vi "Measure vs B2Dv11.vi"() -> ()   [LabVIEW 2009]
doc: "This VI is an example operator panel.\n\nThe VI contains a table for the field values that may be configured manually, or loaded by checking the \"Prompt for File\" box. The data file should contain 3 columns of data, with each column delimited by a tab character.\n\nBefore the VI is executed, set the desired field units and coordinate system. Once the VI is started, follow the directions in the STATUS indicator to operate. Once a field value is achieved, it will be held indefinitely with no user intervention.\n\nThe present field is displayed in the selected units and coordinate system. The present field is queried once per second.\n\nIf a field point is specified that is outside the limits for the magnet, the VI will abort execution."
uses:
  <vilib>/Utility/file.llb/Read From Spreadsheet File (DBL).vi
panel:
  in  "Port Num- TRBridge":string="7"
  in  "GPIB SIM900":string="2"
  in  "TempSensor":bool=TRUE
  in  "AH":bool=TRUE
  in  "GPIB HP 2":string="13"
  in  "Wait between \nVectors":bool
  in  "Change\nPID\n(DetermineSIMPID.vi)":bool
  in  "Wait between \nVectors (ms)":u32=3000
  in  "X Axis":enum16{"B", "phi"}(ring)
  in  "Y Axis":T1(ring)=enum."HP (V)2"
  out "measured data":dbl[][](array[numeric])
  out "XY Graph":T2(graph)
  in  "Notes:":string="Datum: 16.01.12, Uhrzeit: 14:00, Sweep 0.15T/min,(measurevsB2Dv10.vi)), kapazitive Messung, leerer Sensor #1649_1, Referenzmessung, T=0.3K, Winkel 15° , optischer Probenstab, Gestell entfernt" caption="Notizen:"
  out "Messfile Refnum":refnum<file>
  in  "Measurement File":path=path "D:/UserData/Matthias/Messungen/#1649_leer/120116/120116_#1649_135deg_M1.txt"
  in  "Sample name:":string="#1649_1, leer"
  in  "HP 1":bool
  in  "GPIB HP":string="14"
  in  "HP 2":bool
  in  "LI 3":bool
  in  "GPIB L 3":string="8"
  in  "LI 2":bool
  in  "GPIB L 2":string="8"
  in  "LI 1":bool
  in  "GPIB L 1":string="8"
  out "Number of lines":i32=3
  in  "Operation":u16(ring)=1 items=["Stepwise", "Continous"]
  out "Ramp Rate along Vector (T/min)":dbl=0.2123426648592312 format="%.3f"
  out "Current Ramp Rate Z (T/min)":dbl=0.15014787650686168 format="%.3f"
  out "Current Ramp Rate Y (T/min)":dbl=0.15015 format="%.3f"
  in  "User defined Ramp Rate (T/min)":bool=TRUE
  in  "User defined Ramp Rate (T/min)":dbl=0.22 format="%.3f"
  in  "Z-Axis Communications Config":T3={"GPIB address"=22, "GPIB bus"=1, "connection ID"=refnum, "IP"="111.111.111.1", "Active Comm Interface"=0, "Serial Port"="", "Programmer Type"=0} {"Programmer Type" items=["Model 430", "Model 420"]; "Active Comm Interface" items=["TCP/IP (Model 430 Only)", "RS232", "IEEE488"]}
  in  "Max Ramp Rate - Y Axis (A/s)":dbl=0.055 format="%.3f"
  in  "Max Ramp Rate - Z Axis (A/s)":dbl=0.19 format="%.3f"
  in  "Magnitude Limit (kG)":dbl=45.1 format="%.3f"
  in  "Y-Axis Communications Config":T3={"GPIB address"=22, "GPIB bus"=1, "connection ID"=refnum, "IP"="111.111.111.2", "Active Comm Interface"=0, "Serial Port"="", "Programmer Type"=0} {"Programmer Type" items=["Model 430", "Model 420"]; "Active Comm Interface" items=["TCP/IP (Model 430 Only)", "RS232", "IEEE488"]}
  out "Cartesian Display (T)":T4={"Y-Axis Field (T)"=-1e-05, "Z-Axis Field (T)"=2.9999999999999997e-05} {"Z-Axis Field (T)" format="%.3f"; "Y-Axis Field (T)" format="%.3f"}
  in  "Starting index":i32=2
  in  "Normal color":u32(colorbox)=11711154
  in  "Highlight color":u32(colorbox)=16711680
  in  "Prompt for File?":bool
  out "Continue Execution?":bool=TRUE
  out "error out":T5
  in  "error in":T5
  out "STATUS":string="Zeroing vector."
  in  "Ramping Control":u16(ring)=4 items=["NEXT VECTOR", "RAMPING", "HOLDING", "PAUSE", "ZERO"]
  out "Cartesian Display (kG)":T6 {"Z-Axis Field (kG)" format="%.3f"; "Y-Axis Field (kG)" format="%.3f"}
  in  "Field Values":string[][](table)=[["4", "135"], ["-4", "135"], ["0", "0"]]
  out "Switch Heaters":bool=TRUE
  out "Polar Display (T)":T7={"q (degrees)"=315.0, "Field Magnitude (T)"=1.4142135623730951e-05} {"Field Magnitude (T)" format="%.3f"; "q (degrees)" format="%.3f"}
  out "Polar Display (kG)":T8 {"Field Magnitude (kG)" format="%.3f"; "q (degrees)" format="%.3f"}
  in  "Coordinate System":u16(ring)=1 items=["Cartesian", "Polar"]
  in  "Magnetic Field Units":u16(ring)=1 items=["kG", "Tesla"]
  # "kontinuirliche Messung mit PID off bei 0, geht nur im Cartesian mode!"
  # "Measurement Display"
  # "Measurement Settings"
  # "Magnet Settings"
  # "Max Ramp Rate z: 1.27 T/min\nMax Ramp Rate y: 0.17 T/min"
  # "Devices"
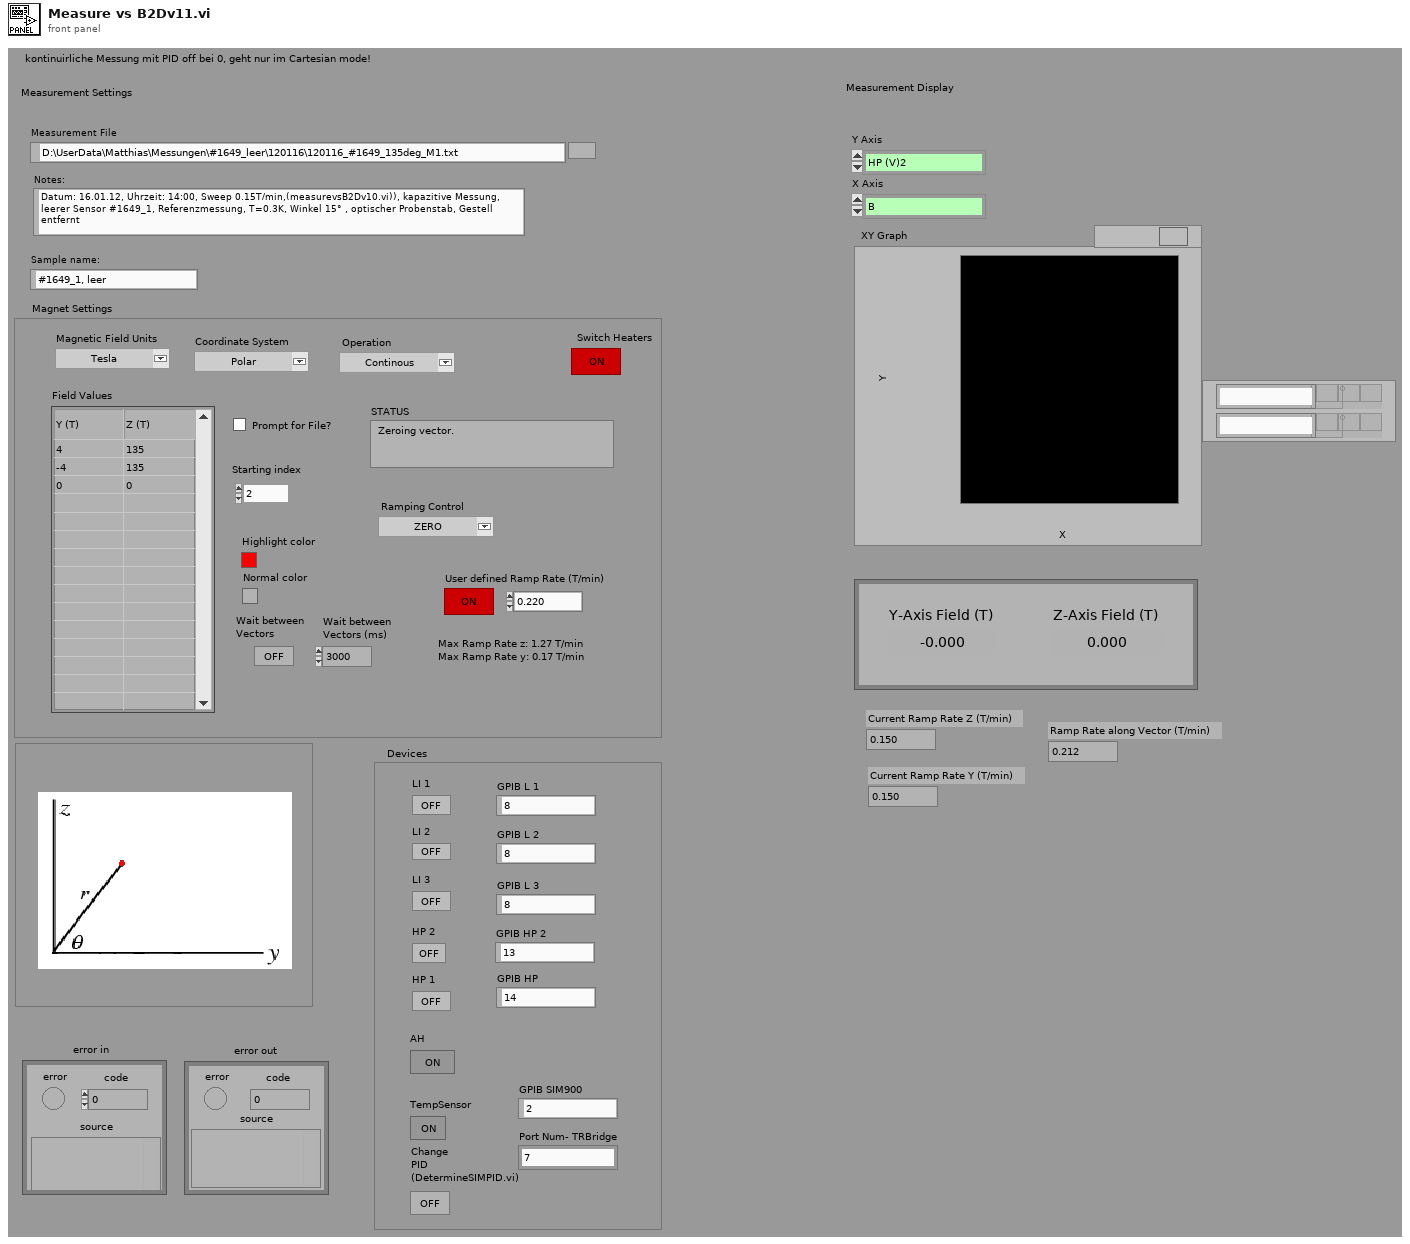
[diagram p1: front panel]
types:
  T1 = enum16{"B", "phi", "LI 1 Vx", "LI 1 Vy", "LI 2 Vx", "LI 2 Vy", "LI 3 Vx", "LI 3 Vy", "LI 4 Vx", "LI 4 Vy", "HP (V)", "HP (V)2", "AH C (pF)", "AH loss"}
  T2 = cluster{"measured data":dbl[], "measured data":dbl[]}
  T3 = cluster{"GPIB address":i16, "GPIB bus":i16, "connection ID":refnum<k5>, "IP":string, "Active Comm Interface":u16, "Serial Port":refnum<visa-resource-name>, "Programmer Type":u16}
  T4 = cluster{"Y-Axis Field (T)":dbl, "Z-Axis Field (T)":dbl}
  T5 = cluster{"error":bool, "code":i32, "source":string}
  T6 = cluster{"Y-Axis Field (kG)":dbl, "Z-Axis Field (kG)":dbl}
  T7 = cluster{"q (degrees)":dbl, "Field Magnitude (T)":dbl}
  T8 = cluster{"q (degrees)":dbl, "Field Magnitude (kG)":dbl}
  T9 = enum16{"", "RAMPING", "HOLDING", "PAUSED", "MANUAL UP", "MANUAL DOWN", "ZEROING CURRENT", "QUENCH DETECTED", "HEATING SWITCH"}
  T10 = enum16{"", "RAMPING", "HOLDING", "PAUSED", "MANUAL UP", "MANUAL DOWN", "ZEROING CURRENT", "QUENCH DETECTED", "HEATING SWITCH", "AT ZER0", "COOLING SWITCH"}
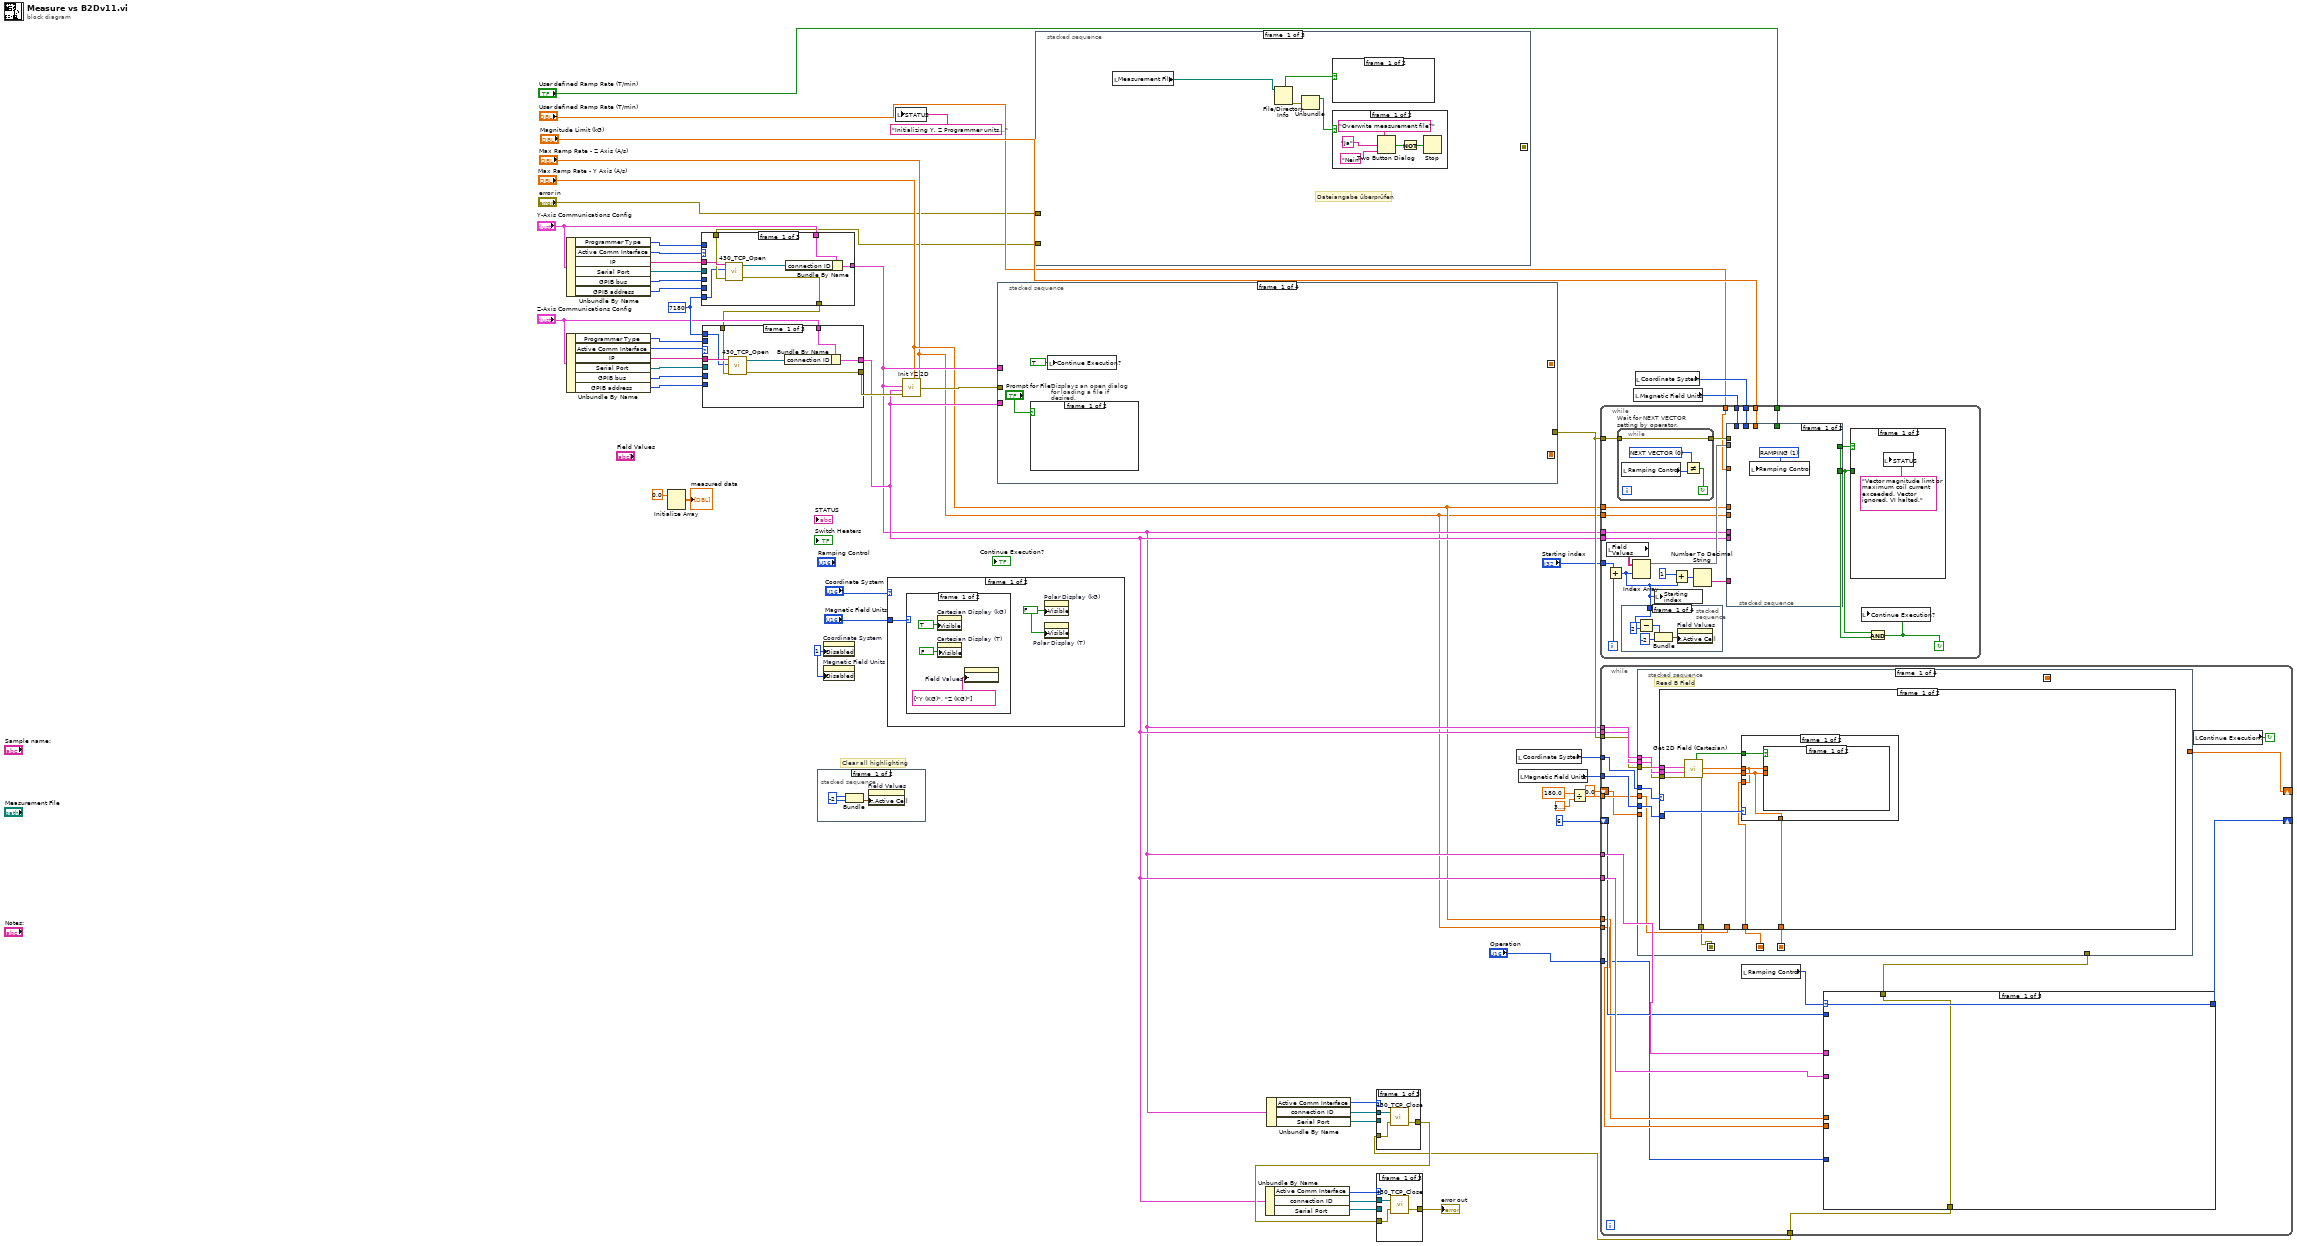
[diagram p0: block diagram]
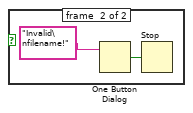
[diagram p3: hidden frame]
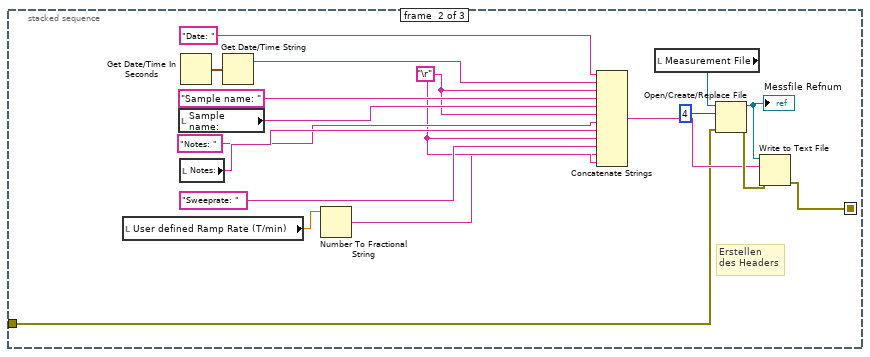
[diagram p4: hidden frame]
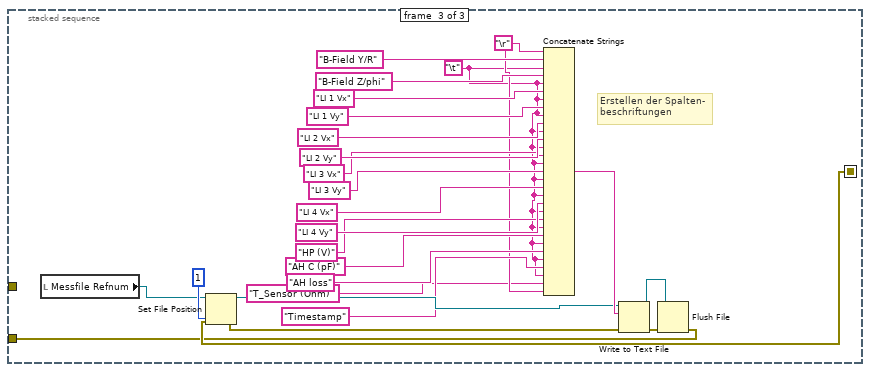
[diagram p5: hidden frame]
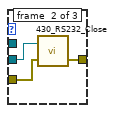
[diagram p6: hidden frame]
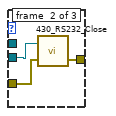
[diagram p8: hidden frame]
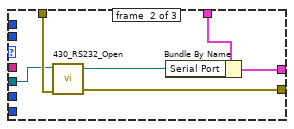
[diagram p10: hidden frame]
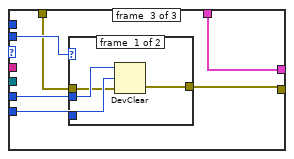
[diagram p11: hidden frame]
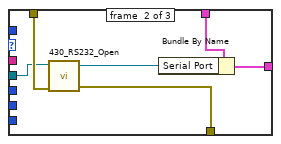
[diagram p13: hidden frame]
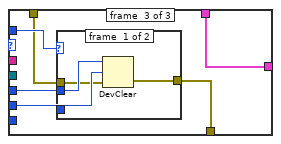
[diagram p14: hidden frame]
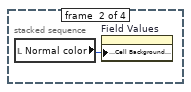
[diagram p16: hidden frame]
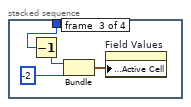
[diagram p17: hidden frame]
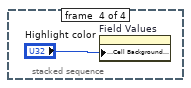
[diagram p18: hidden frame]
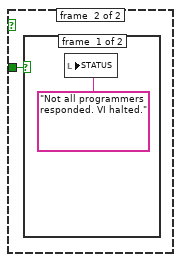
[diagram p19: hidden frame]
diagram:
  w39 = 7180 ("TCP Port")
  w52 = u8 1 ("Write Attribute")
  # "Clear all highlighting"
  n1 = Unbundle By Name("Z-Axis Communications Config") -> ("Programmer Type"=w15:u16, "Active Comm Interface"=w38:u16, "IP"=w35:string, "Serial Port"=w34:refnum<visa-resource-name>, "GPIB bus"=w14:i16, "GPIB address"=w13:i16)
  n2 = Unbundle By Name("Y-Axis Communications Config") -> ("Programmer Type"=w9:u16, "Active Comm Interface"=w37:u16, "IP"=w36:string, "Serial Port"=w33:refnum<visa-resource-name>, "GPIB bus"=w10:i16, "GPIB address"=w11:i16)
  n3 = Initialize Array(0.0 ("element")) -> (→"measured data":dbl[][])  [unwired: 2 in]
  n4 = stacked-sequence {
    frame #0 {
      w55 = -2
      n5 = Bundle(w55, w55) -> (w56:cluster{i32, i32})  [unwired: 1 in]
      n6 = property on="Field Values" class="Tbl (strict)"("Active Cell:Active Cell"=w56) -> ()  [unwired: 2 in, 2 out]
    }
    frame #1 {
      n7 = property on="Field Values" class="Tbl (strict)"("Active Cell:Cell Background Color"="Normal color") -> ()  [unwired: 2 in, 2 out]
    }
  }
  n8 = property on="Coordinate System" class="Ring (strict)"("Disabled"=w52) -> ()  [unwired: 2 in, 2 out]
  n9 = property on="Magnetic Field Units" class="Ring (strict)"("Disabled"=w52) -> ()  [unwired: 2 in, 2 out]
  n10 = case shown="0, Default" "Coordinate System" {
    tunnel: "Magnetic Field Units" -> [w59 w67]
    frame #0 {
      w58 = FALSE ("Write Attribute")
      (unwired) FALSE ("Write Attribute")
      (unwired) TRUE ("Write Attribute")
      n11 = case shown="1" w59 {
        frame #0 {
          n12 = property on="Cartesian Display (kG)" class="Cluster (strict)"("Visible"=TRUE ("Write Attribute")) -> ()  [unwired: 2 in, 2 out]
          n13 = property on="Cartesian Display (T)" class="Cluster (strict)"("Visible"=FALSE ("Write Attribute")) -> ()  [unwired: 2 in, 2 out]
          n14 = property on="Field Values" class="Tbl (strict)"("Column Header Strings[]"=string[] ["Y (KG)", "Z (KG)"] ("Write Attribute")) -> ()  [unwired: 2 in, 2 out]
        }
        frame #1 {
          n15 = property on="Cartesian Display (kG)" class="Cluster (strict)"("Visible"=FALSE ("Write Attribute")) -> ()  [unwired: 2 in, 2 out]
          n16 = property on="Cartesian Display (T)" class="Cluster (strict)"("Visible"=TRUE ("Write Attribute")) -> ()  [unwired: 2 in, 2 out]
          n17 = property on="Field Values" class="Tbl (strict)"("Column Header Strings[]"=string[] ["Y (T)", "Z (T)"] ("Write Attribute")) -> ()  [unwired: 2 in, 2 out]
        }
      }
      n18 = property on="Polar Display (kG)" class="Clust (strict)"("Visible"=w58) -> ()  [unwired: 2 in, 2 out]
      n19 = property on="Polar Display (T)" class="Clust (strict)"("Visible"=w58) -> ()  [unwired: 2 in, 2 out]
    }
    frame #1 {
      (unwired) FALSE ("Write Attribute")
      (unwired) TRUE ("Write Attribute")
      w66 = FALSE ("Write Attribute")
      n20 = case shown="1" w67 {
        frame #0 {
          n21 = property on="Polar Display (kG)" class="Clust (strict)"("Visible"=TRUE ("Write Attribute")) -> ()  [unwired: 2 in, 2 out]
          n22 = property on="Polar Display (T)" class="Clust (strict)"("Visible"=FALSE ("Write Attribute")) -> ()  [unwired: 2 in, 2 out]
          n23 = property on="Field Values" class="Tbl (strict)"("Column Header Strings[]"=string[] ["Mag. r (KG)", "Theta (deg)"] ("Write Attribute")) -> ()  [unwired: 2 in, 2 out]
        }
        frame #1 {
          n24 = property on="Polar Display (kG)" class="Clust (strict)"("Visible"=FALSE ("Write Attribute")) -> ()  [unwired: 2 in, 2 out]
          n25 = property on="Polar Display (T)" class="Clust (strict)"("Visible"=TRUE ("Write Attribute")) -> ()  [unwired: 2 in, 2 out]
          n26 = property on="Field Values" class="Tbl (strict)"("Column Header Strings[]"=string[] ["Mag. r (T)", "Theta (deg)"] ("Write Attribute")) -> ()  [unwired: 2 in, 2 out]
        }
      }
      n27 = property on="Cartesian Display (kG)" class="Cluster (strict)"("Visible"=w66) -> ()  [unwired: 2 in, 2 out]
      n28 = property on="Cartesian Display (T)" class="Cluster (strict)"("Visible"=w66) -> ()  [unwired: 2 in, 2 out]
    }
  }
  n29 = local write "STATUS"("Initializing Y, Z Programmer units..." ("STATUS")) -> ()
  n30 = stacked-sequence {
    seq-local: [_ w85 _] -> [_ _ w110]
    tunnel: "error in" -> [_ w86 _]
    tunnel: [_ _ w109] -> w4
    frame #0 {
      # "Dateiangabe überprüfen"
      n31 = local read "Measurement File"() -> (w77:path)
      n32 = File/Directory Info(path=w77) -> (directory=w75:bool, error out=w76:errorcluster)  [unwired: 1 in, 5 out]
      n33 = Unbundle(w76) -> ("status"=w74:bool)  [unwired: 2 out]
      n34 = case shown="False" w75 {
        frame #0 {
        }
        frame #1 {
          n35 = One Button Dialog(message="Invalid\nfilename!") -> (true=w83:bool)  [unwired: 1 in]
          n36 = Stop(stop? (T)=w83) -> ()
        }
      }
      n37 = case shown="False" w74 {
        frame #0 {
          n38 = Two Button Dialog(message="Overwrite measurement file?", 1:"Nein", 2:"Ja") -> (T button?=w79:bool)
          n39 = Not(x=w79) -> (.not. x?=w78:bool)
          n40 = Stop(stop? (T)=w78) -> ()
        }
        frame #1 {
        }
      }
    }
    frame #1 {
      w89 = "\r"
      # "Erstellen\ndes Headers"
      n41 = local read "User defined Ramp Rate (T/min)"() -> (w88:dbl)
      n42 = local read "Sample name:"() -> (w95:string)
      n43 = local read "Notes:"() -> (w97:string)
      n44 = Get Date/Time In Seconds() -> (seconds since 1Jan1904=w91:timestamp)
      n45 = Get Date/Time String(seconds (now)=w91) -> (date string=w93:string)  [unwired: 2 in, 1 out]
      n46 = Number To Fractional String(number=w88) -> (F-format string=w87:string)  [unwired: 3 in]
      n47 = Concatenate Strings("Date: ", w93, w89, "Sample name: ", w95, w89, "Notes: ", w97, w89, "Sweeprate: ", w87, w89) -> (w101:string)
      n48 = local read "Measurement File"() -> (w98:path)
      n49 = Open/Create/Replace File(file path (use dialog)=w98, error in=w86, operation (0:open)=4) -> (refnum out=w100:refnum<file>, error out=w102:errorcluster)  [unwired: 3 in, 1 out]
      "Messfile Refnum" <- w100
      n50 = Write to Text File(file (use dialog)=w100, text=w101, error in=w102) -> (error out=w85:errorcluster)  [unwired: 1 in, 2 out]
    }
    frame #2 {
      w104 = "\t"
      w105 = "\r"
      # "Erstellen der Spalten-\nbeschriftungen"
      n51 = local read "Messfile Refnum"() -> (w117:refnum<file>)
      n52 = Set File Position(refnum=w117, from (0:start)=1, error in=w110) -> (refnum out=w123:refnum<file>, error out=w125:errorcluster)  [unwired: 1 in]
      n53 = Concatenate Strings(w105, "B-Field Y/R", w104, "B-Field Z/phi", w104, "LI 1 Vx", w104, "LI 1 Vy", w104, "LI 2 Vx", w104, "LI 2 Vy", w104, "LI 3 Vx", w104, "LI 3 Vy", w104, "LI 4 Vx", w104, "LI 4 Vy", w104, "HP (V)", w104, "AH C (pF)" ("string"), w104, "AH loss" ("string"), w104, "Timestamp", w104, "T_Sensor (Ohm)" ("string"), w105) -> (w124:string)
      n54 = Write to Text File(file (use dialog)=w123, text=w124, error in=w125) -> (refnum out=w127:refnum<file>, error out=w126:errorcluster)  [unwired: 1 in, 1 out]
      n55 = Flush File(refnum=w127, error in=w126) -> (error out=w109:errorcluster)  [unwired: 1 out]
    }
  }
  n56 = case shown="0, Default" w37 {
    tunnel: w36 -> [w135 _ _]
    tunnel: w4 -> [w134 w141 w143]
    tunnel: "Y-Axis Communications Config" -> [w133 w136 w147]
    tunnel: [w131 w139 w147] -> w22
    tunnel: [w130 w140 w142] -> w12
    tunnel: w39 -> [w129 _ _]
    tunnel: w33 -> [_ w137 _]
    tunnel: w11 -> [_ _ w146]
    tunnel: w10 -> [_ _ w145]
    tunnel: w9 -> [_ _ w144]
    frame #0 {
      n57 = call <userlib>:"430_TCP_Open.vi"("IP Address"=w135, "TCP Port"=w129, "error in (no error)"=w134) -> ("connection ID"=w132:refnum<k5>, "error out"=w130:errorcluster)  [unwired: 3 in, 1 out]
      n58 = Bundle By Name(cluster=w133, "connection ID"=w132) -> (w131:T3)
    }
    frame #1 {
      n59 = call <userlib>:"430_RS232_Open.vi"("VISA resource name"=w137, "error in (no error)"=w141) -> ("VISA resource name out"=w138:refnum<visa-resource-name>, "error out"=w140:errorcluster)  [unwired: 5 in]
      n60 = Bundle By Name(cluster=w136, "Serial Port"=w138) -> (w139:T3)
    }
    frame #2 {
      n61 = case shown="1" w144 {
        tunnel: w145 -> [w151 _]
        tunnel: w146 -> [w150 _]
        tunnel: w143 -> [w149 w152]
        tunnel: [w148 w152] -> w142
        frame #0 {
          n62 = DevClear(2:w149, 3:w150, 4:w151) -> (0:w148:errorcluster)  [unwired: 1 out]
        }
        frame #1 {
        }
      }
    }
  }
  n63 = case shown="0, Default" w38 {
    tunnel: w35 -> [w159 _ _]
    tunnel: w12 -> [w158 w165 w167]
    tunnel: [w157 w164 w166] -> w32
    tunnel: "Z-Axis Communications Config" -> [w156 w162 w171]
    tunnel: [w154 w163 w171] -> w23
    tunnel: w39 -> [w153 _ _]
    tunnel: w34 -> [_ w160 _]
    tunnel: w15 -> [_ _ w170]
    tunnel: w14 -> [_ _ w169]
    tunnel: w13 -> [_ _ w168]
    frame #0 {
      n64 = call <userlib>:"430_TCP_Open.vi"("IP Address"=w159, "TCP Port"=w153, "error in (no error)"=w158) -> ("connection ID"=w155:refnum<k5>, "error out"=w157:errorcluster)  [unwired: 3 in, 1 out]
      n65 = Bundle By Name(cluster=w156, "connection ID"=w155) -> (w154:T3)
    }
    frame #1 {
      n66 = call <userlib>:"430_RS232_Open.vi"("VISA resource name"=w160, "error in (no error)"=w165) -> ("VISA resource name out"=w161:refnum<visa-resource-name>, "error out"=w164:errorcluster)  [unwired: 5 in]
      n67 = Bundle By Name(cluster=w162, "Serial Port"=w161) -> (w163:T3)
    }
    frame #2 {
      n68 = case shown="0, Default" w170 {
        tunnel: w169 -> [w175 _]
        tunnel: w168 -> [w174 _]
        tunnel: w167 -> [w173 w176]
        tunnel: [w172 w176] -> w166
        frame #0 {
          n69 = DevClear(2:w173, 3:w174, 4:w175) -> (0:w172:errorcluster)  [unwired: 1 out]
        }
        frame #1 {
        }
      }
    }
  }
  n70 = call <userlib>:"Init YZ 2D.vi"("Max Ramp Rate Z-axis"="Max Ramp Rate - Z Axis (A/s)", "Max Ramp Rate Y-axis"="Max Ramp Rate - Y Axis (A/s)", "error in"=w32, "Z-Axis Communications Config"=w23, "Y-Axis Communications Config"=w22) -> ("error out"=w50:T5)  [unwired: 5 in]
  n71 = stacked-sequence {
    seq-local: [_ w184 _ _] -> [_ _ w231 _]
    seq-local: [_ w183 _ _] -> [_ _ w230 _]
    tunnel: w23 -> [_ w186 _ _]
    tunnel: w50 -> [_ w187 _ _]
    tunnel: [_ w182 _ _] -> w46
    tunnel: w22 -> [_ w185 _ _]
    frame #0 {
      n72 = case "Displays an open dialog for loading a file if desired." shown="True" "Prompt for File?" {
        frame #0 {
        }
        frame #1 {
          n73 = call-poly <vilib>:"Read From Spreadsheet File.vi"() -> ("all rows"=w181:dbl[][])  [unwired: 7 in, 4 out]
          n74 = Number To Fractional String(number=w181, precision (6)=i16 4) -> (F-format string=w180:string[][])  [unwired: 2 in]
          n75 = local write "Field Values"(w180) -> ()
        }
      }
      n76 = local write "Continue Execution?"(TRUE ("Continue Execution?")) -> ()
    }
    frame #1 {
      w195 = u16 3 items=["NEXT VECTOR", "RAMPING", "HOLDING", "PAUSE", "ZERO"] ("Ramping Control")
      n77 = call <userlib>:"Get Switch Present.vi"("error in"=w187, "Communications Config"=w185) -> ("error out"=w191:T5, "Switch Present?"=w192:bool)
      n78 = case shown="True" w192 {
        tunnel: w191 -> [w213 w222]
        tunnel: w185 -> [_ w215]
        tunnel: [0.0 w219] -> w183
        tunnel: [w213 w221] -> w190
        frame #0 {
        }
        frame #1 {
          n79 = call <userlib>:"Get Switch Heater Time.vi"("error in"=w222, "Communications Config"=w215) -> ("error out"=w218:T5, "Switch Heating Time (secs)"=w220:dbl)
          n80 = call <userlib>:"Get Switch Heater.vi"("error in"=w218, "Communications Config"=w215) -> ("error out"=w217:T5, "Switch Heater Indicator"=w216:bool)
          n81 = case shown="False" w216 {
            tunnel: [w227 w228] -> w221
            tunnel: w220 -> [w225 _]
            tunnel: [w225 0.0] -> w219
            tunnel: w217 -> [w223 w228]
            tunnel: w215 -> [w224 _]
            frame #0 {
              n82 = call <userlib>:"Set Switch Heater.vi"("error in"=w223, "Switch Heater Control"=TRUE, "Communications Config"=w224) -> ("error out"=w227:T5)
            }
            frame #1 {
            }
          }
        }
      }
      n83 = call <userlib>:"Get Switch Present.vi"("error in"=w190, "Communications Config"=w186) -> ("error out"=w188:T5, "Switch Present?"=w189:bool)
      n84 = case shown="True" w189 {
        tunnel: w188 -> [w196 w205]
        tunnel: w186 -> [_ w198]
        tunnel: [0.0 w202] -> w184
        tunnel: [w196 w204] -> w182
        frame #0 {
        }
        frame #1 {
          n85 = call <userlib>:"Get Switch Heater Time.vi"("error in"=w205, "Communications Config"=w198) -> ("error out"=w201:T5, "Switch Heating Time (secs)"=w203:dbl)
          n86 = call <userlib>:"Get Switch Heater.vi"("error in"=w201, "Communications Config"=w198) -> ("error out"=w200:T5, "Switch Heater Indicator"=w199:bool)
          n87 = case shown="False" w199 {
            tunnel: [w206 w211] -> w204
            tunnel: w203 -> [w209 _]
            tunnel: [w209 0.0] -> w202
            tunnel: w200 -> [w207 w211]
            tunnel: w198 -> [w208 _]
            frame #0 {
              n88 = call <userlib>:"Set Switch Heater.vi"("error in"=w207, "Switch Heater Control"=TRUE, "Communications Config"=w208) -> ("error out"=w206:T5)
            }
            frame #1 {
            }
          }
        }
      }
      n89 = local write "Ramping Control"(w195) -> ()
      n90 = local write "Switch Heaters"(TRUE ("Switch Heater Control")) -> ()
      n91 = property on="Switch Heaters" class="Boolean (strict)"("Disabled"=u8 1 ("Write Attribute")) -> ()  [unwired: 2 in, 2 out]
    }
    frame #2 {
      n92 = Max & Min(x=w231, y=w230) -> (max(x,y)=w232:dbl)  [unwired: 1 out]
      n93 = local write "STATUS"("Heating switches..." ("STATUS")) -> ()
      n94 = Add(x=w232, y=2) -> (x+y=w236:dbl)
      n95 = property on="Ramping Control" class="Ring (strict)"("Disabled"=u8 1 ("Write Attribute")) -> ()  [unwired: 2 in, 2 out]
      n96 = Multiply(x=w236, y=1000) -> (x*y=w235:dbl)
      n97 = Wait (ms)(milliseconds to wait=w235) -> ()  [unwired: 1 out]
    }
    frame #3 {
      n98 = property on="Ramping Control" class="Ring (strict)"("Disabled"=u8 0 ("Write Attribute")) -> ()  [unwired: 2 in, 2 out]
      n99 = local write "STATUS"("Ready to ramp to first vector. Set Ramping Mode to NEXT VECTOR to begin." ("STATUS")) -> ()
      n100 = local read "Field Values"() -> (w241:string[][])
      n101 = Array Size(array=w241) -> (size(s)=w240:i32[])
      n102 = Index Array(array=w240, index=0) -> (element=→"Number of lines":i32)
    }
  }
  n103 = Unbundle By Name(w23) -> ("Active Comm Interface"=w29:u16, "connection ID"=w28:refnum<k5>, "Serial Port"=w27:refnum<visa-resource-name>)
  n104 = Unbundle By Name(w22) -> ("Active Comm Interface"=w30:u16, "connection ID"=w26:refnum<k5>, "Serial Port"=w25:refnum<visa-resource-name>)
  n105 = local read "Coordinate System"() -> (w47:u16)
  n106 = local read "Magnetic Field Units"() -> (w45:u16)
  n107 = Divide(x=180.0, y=3.141592653589793) -> (x/y=w42:dbl)
  n108 = while {
    shift-left: u16 6 ("Ramping Control") -> [w251]
    shift-right: [w252] -> _
    tunnel: [w254] -> w24
    tunnel: w23 -> [w255]
    tunnel: w22 -> [w256]
    tunnel: w42 -> [w258]
    tunnel: w45 -> [w259]
    tunnel: w46 -> [w260]
    tunnel: w23 -> [w261]
    tunnel: w22 -> [w262]
    tunnel: w47 -> [w263]
    tunnel: "Max Ramp Rate - Y Axis (A/s)" -> [w250]
    tunnel: "Max Ramp Rate - Z Axis (A/s)" -> [w249]
    tunnel: "Operation" -> [w248]
    shift-right: [w246] -> _
    shift-left: 0.0 -> [w245]
    stop <- w253 continue-if-true
    n109 = stacked-sequence {
      seq-local: [w266 _ _ _] -> [_ _ w391 _]
      seq-local: [w265 _ _ _] -> [_ w339 w388 _]
      seq-local: [w264 _ _ _] -> [_ w340 w389 _]
      seq-local: [_ _ w376 _] -> [_ _ _ w468]
      tunnel: w263 -> [w272 _ _ w466]
      tunnel: w262 -> [w271 _ _ _]
      tunnel: w261 -> [w270 _ _ _]
      tunnel: w260 -> [w269 _ _ _]
      tunnel: w259 -> [w268 _ _ _]
      tunnel: w258 -> [w267 _ _ _]
      tunnel: [_ _ w390 _] -> w247
      tunnel: [_ w342 _ _] -> w246
      tunnel: w245 -> [_ w341 _ _]
      frame #0 {
        # "Read B Field"
        n110 = case shown="0, Default" w272 {
          tunnel: w271 -> [w282 w305]
          tunnel: w270 -> [w281 w304]
          tunnel: w269 -> [w280 w303]
          tunnel: w268 -> [w279 w302]
          tunnel: w267 -> [_ w301]
          tunnel: [w275 w300] -> w266
          tunnel: [w274 w298] -> w265
          tunnel: [w273 w299] -> w264
          frame #0 {
            n111 = call <userlib>:"Get 2D Field (Cartesian).vi"("Y-Axis Communications Config"=w282, "Z-Axis Communications Config"=w281, "error in"=w280) -> ("All Instruments Responded?"=w276:bool, "Y-Axis Field (kG)"=w278:dbl, "Z-Axis Field (kG)"=w277:dbl, "error out"=w275:T5)  [unwired: 2 in]
            n112 = case shown="0, Default" w279 {
              tunnel: w278 -> [w283 w291]
              tunnel: w277 -> [w284 w292]
              tunnel: w276 -> [w285 w294]
              tunnel: [w284 w290] -> w274
              tunnel: [w283 w289] -> w273
              frame #0 {
                n113 = case shown="True" w285 {
                  tunnel: w283 -> [_ w287]
                  tunnel: w284 -> [_ w286]
                  frame #0 {
                  }
                  frame #1 {
                    n114 = Bundle("Y-Axis Field (kG)"=w287, "Z-Axis Field (kG)"=w286) -> (→"Cartesian Display (kG)":T6)  [unwired: 1 in]
                  }
                }
              }
              frame #1 {
                w293 = 0.1 ("y")
                n115 = Multiply(x=w291, y=w293) -> (x*y=w289:dbl)
                n116 = Multiply(x=w292, y=w293) -> (x*y=w290:dbl)
                n117 = case shown="True" w294 {
                  tunnel: w289 -> [_ w297]
                  tunnel: w290 -> [_ w296]
                  frame #0 {
                  }
                  frame #1 {
                    n118 = Bundle(w297, w296) -> (→"Cartesian Display (T)":cluster{dbl, dbl})  [unwired: 1 in]
                  }
                }
              }
            }
          }
          frame #1 {
            n119 = stacked-sequence {
              tunnel: w305 -> [w316]
              tunnel: w304 -> [w315]
              tunnel: w303 -> [w314]
              tunnel: w302 -> [w313]
              tunnel: w301 -> [w310]
              tunnel: [w308] -> w300
              tunnel: [w307] -> w298
              tunnel: [w306] -> w299
              frame #0 {
                # "Field"
                n120 = call <userlib>:"Get 2D Field (Polar).vi"("Y-Axis Communications Config"=w316, "Z-Axis Communications Config"=w315, "error in"=w314) -> ("All Instruments Responded?"=w309:bool, "Radial (r) Field (kG)"=w312:dbl, "q (radians)"=w311:dbl, "error out"=w308:T5)  [unwired: 2 in]
                n121 = case shown="1" w313 {
                  tunnel: w312 -> [w318 w330]
                  tunnel: w311 -> [w320 w329]
                  tunnel: w310 -> [w319 w328]
                  tunnel: w309 -> [w321 w327]
                  tunnel: [w318 w325] -> w307
                  tunnel: [w317 w326] -> w306
                  frame #0 {
                    n122 = Multiply(x=w320, y=w319) -> (x*y=w317:dbl)
                    n123 = case shown="True" w321 {
                      tunnel: w318 -> [_ w322]
                      tunnel: w317 -> [_ w323]
                      frame #0 {
                      }
                      frame #1 {
                        n124 = Bundle(w323, "Radial (r) Field (kG)"=w322) -> (→"Polar Display (kG)":cluster{dbl, "Radial (r) Field (kG)":dbl})  [unwired: 1 in]
                      }
                    }
                  }
                  frame #1 {
                    n125 = Multiply(x=w330, y=0.1) -> (x*y=w326:dbl)
                    n126 = Multiply(x=w329, y=w328) -> (x*y=w325:dbl)
                    n127 = case shown="True" w327 {
                      tunnel: w326 -> [_ w332]
                      tunnel: w325 -> [_ w333]
                      frame #0 {
                      }
                      frame #1 {
                        n128 = Bundle(w333, w332) -> (→"Polar Display (T)":cluster{dbl, dbl})  [unwired: 1 in]
                      }
                    }
                  }
                }
              }
            }
          }
        }
      }
      frame #1 {
        # "Change PID"
        n129 = Square(x=w340) -> (x^2=w337:dbl)
        n130 = Square(x=w339) -> (x^2=w338:dbl)
        n131 = Add(x=w337, y=w338) -> (x+y=w336:dbl)
        n132 = Square Root(x=w336) -> (sqrt(x)=w335:dbl)
        n133 = case shown="True" "Change\nPID\n(DetermineSIMPID.vi)" {
          tunnel: w335 -> [_ w354]
          tunnel: [_ w350] -> w342
          tunnel: w341 -> [_ w352]
          frame #0 {
          }
          frame #1 {
            n134 = Absolute Value(x=w354) -> (abs(x)=w350:dbl)
            n135 = Less Or Equal?(x=w350, y=0.07 ("upper limit")) -> (x <= y?=w347:bool)
            n136 = Greater?(x=w352, y=0.07 ("upper limit")) -> (0:w348:bool)
            n137 = Not(x=w348) -> (.not. x?=w345:bool)
            n138 = Not(x=w347) -> (.not. x?=w346:bool)
            n139 = And(x=w348, y=w347) -> (x .and. y?=w353:bool)
            n140 = And(x=w345, y=w346) -> (x .and. y?=w344:bool)
            n141 = case shown="True" w353 {
              frame #0 {
              }
              frame #1 {
                n142 = stacked-sequence {
                  frame #0 {
                    n143 = call "SIM960Poff.vi"("off/on (0/1)"="0", "Port Num- PID"="1", "GPIB-Adress"="2") -> ()  [unwired: 9 in]
                  }
                  frame #1 {
                    n144 = call "SIM960Poff.vi"("off/on (0/1)"="0", "Port Num- PID"="3", "GPIB-Adress"="2") -> ()  [unwired: 9 in]
                  }
                  frame #2 {
                    n145 = call "SIM960ChangeSignP.vi"("Port Num- PID"="1", "GPIB-Adress"="2") -> ()  [unwired: 10 in]
                  }
                }
              }
            }
            n146 = case shown="True" w344 {
              frame #0 {
              }
              frame #1 {
                n147 = stacked-sequence {
                  frame #0 {
                    n148 = call "SIM960Poff.vi"("off/on (0/1)"="1", "Port Num- PID"="3", "GPIB-Adress"="2") -> ()  [unwired: 9 in]
                  }
                  frame #1 {
                    n149 = call "SIM960Poff.vi"("off/on (0/1)"="1", "Port Num- PID"="1", "GPIB-Adress"="2") -> ()  [unwired: 9 in]
                  }
                }
              }
            }
          }
        }
      }
      frame #2 {
        w375 = u16 2 items=["NEXT VECTOR", "RAMPING", "HOLDING", "PAUSE", "ZERO"] ("Ramping Control")
        # "Zeile in Datei schreiben"
        # "Read and Save Devices"
        n150 = stacked-sequence {
          tunnel: [w403 _ _ _ _ _ _ _] -> w387
          tunnel: [w402 _ _ _ _ _ _ _] -> w386
          tunnel: [_ w416 _ _ _ _ _ _] -> w383
          tunnel: [_ w414 _ _ _ _ _ _] -> w382
          tunnel: [_ _ w426 _ _ _ _ _] -> w381
          tunnel: [_ _ w425 _ _ _ _ _] -> w380
          tunnel: [_ _ _ w437 _ _ _ _] -> w379
          tunnel: [_ _ _ 0.0 _ _ _ _] -> w378
          tunnel: [_ _ _ _ w443 _ _ _] -> w377
          tunnel: [_ _ _ _ _ _ _ w462] -> w370
          tunnel: [_ _ _ _ _ w450 _ _] -> w372
          tunnel: [_ _ _ _ _ w449 _ _] -> w371
          tunnel: [_ _ _ _ _ _ w455 _] -> w369
          frame #0 {
            n151 = case shown="True" "LI 1" {
              tunnel: ["0" ("Antwort2") w410] -> w405
              tunnel: ["0" ("Antwort1") w409] -> w404
              frame #0 {
              }
              frame #1 {
                n152 = call "LI-Ansteuerung.vi"("Frage2"="OUTP? 2", "Frage1"="OUTP? 1", "address string"="GPIB L 1") -> ("Antwort2"=w410:string, "Antwort1"=w409:string)
              }
            }
            n153 = Fract/Exp String To Number(string=w405) -> (number=w402:dbl)  [unwired: 3 in, 1 out]
            n154 = Fract/Exp String To Number(string=w404) -> (number=w403:dbl)  [unwired: 3 in, 1 out]
          }
          frame #1 {
            n155 = case shown="True" "LI 2" {
              tunnel: [w419 w421] -> w415
              tunnel: [w419 w420] -> w417
              frame #0 {
                w419 = "0" ("Antwort1")
              }
              frame #1 {
                n156 = call "LI-Ansteuerung.vi"("Frage2"="OUTP? 2", "Frage1"="OUTP? 1", "address string"="GPIB L 2") -> ("Antwort2"=w421:string, "Antwort1"=w420:string)
              }
            }
            n157 = Fract/Exp String To Number(string=w415) -> (number=w414:dbl)  [unwired: 3 in, 1 out]
            n158 = Fract/Exp String To Number(string=w417) -> (number=w416:dbl)  [unwired: 3 in, 1 out]
          }
          frame #2 {
            n159 = case shown="True" "LI 3" {
              tunnel: [w430 w432] -> w427
              tunnel: [w430 w431] -> w428
              frame #0 {
                w430 = "0" ("Antwort1")
              }
              frame #1 {
                n160 = call "LI-Ansteuerung.vi"("Frage2"="OUTP? 2", "Frage1"="OUTP? 1", "address string"="GPIB L 3") -> ("Antwort2"=w432:string, "Antwort1"=w431:string)
              }
            }
            n161 = Fract/Exp String To Number(string=w428) -> (number=w426:dbl)  [unwired: 3 in, 1 out]
            n162 = Fract/Exp String To Number(string=w427) -> (number=w425:dbl)  [unwired: 3 in, 1 out]
          }
          frame #3 {
            n163 = case shown="False" "HP 2" {
              tunnel: [0.0 ("Voltage") w440] -> w437
              frame #0 {
              }
              frame #1 {
                n164 = call "HP-ReadVoltagev2.vi"("String"="meas:volt:dc? 10,0.001", "HP-Mulitmeter\nGPIB Address"="GPIB HP 2") -> ("Voltage"=w440:dbl)  [unwired: 9 in]
              }
            }
          }
          frame #4 {
            n165 = case shown="False" "HP 1" {
              tunnel: [0.0 ("Voltage") w447] -> w443
              frame #0 {
              }
              frame #1 {
                n166 = call "HP-ReadVoltagev2.vi"("String"="meas:volt:dc? 200,0.001", "HP-Mulitmeter\nGPIB Address"="GPIB HP") -> ("Voltage"=w447:dbl)  [unwired: 9 in]
              }
            }
          }
          frame #5 {
            n167 = case shown="True" "AH" {
              tunnel: [w452 w454] -> w449
              tunnel: [w452 w453] -> w450
              frame #0 {
                w452 = 0.0 ("Voltage")
              }
              frame #1 {
                n168 = call "AHRead2.vi"() -> ("loss"=w454:dbl, "capacitance"=w453:dbl)  [unwired: 8 in, 2 out]
              }
            }
          }
          frame #6 {
            n169 = case shown="False" "TempSensor" {
              tunnel: [0.0 ("Voltage") w458] -> w455
              frame #0 {
              }
              frame #1 {
                n170 = call "Read_R_Bridge_new_v3.vi"("Port Num- TRBridge"="Port Num- TRBridge", "GPIB-Adress"="GPIB SIM900") -> ("R out"=w459:string)  [unwired: 8 in, 1 out]
                n171 = Fract/Exp String To Number(string=w459) -> (number=w458:dbl)  [unwired: 3 in, 1 out]
              }
            }
          }
          frame #7 {
            n172 = Get Date/Time In Seconds() -> (seconds since 1Jan1904=w463:timestamp)
            n173 = To Double Precision Float(number=w463) -> (double precision float=w462:dbl)
          }
        }
        n174 = local read "Ramping Control"() -> (w374:u16)
        n175 = Build Array(w389, w388, w387, w386, w383, w382, w380, w381, w379, w378, w377, w372, w371, w369, w370) -> (w376:dbl[])
        n176 = Array To Spreadsheet String(array=w376, 3:"%.8f" ("format string")) -> (spreadsheet string=w385:string)  [unwired: 1 in]
        n177 = Equal?(x=w374, y=w375) -> (x = y?=w373:bool)
        n178 = case shown="False" w373 {
          tunnel: w391 -> [w400 w401]
          tunnel: [w399 w401] -> w390
          tunnel: w385 -> [w398 _]
          frame #0 {
            n179 = local read "Messfile Refnum"() -> (w392:refnum<file>)
            n180 = Set File Position(refnum=w392, from (0:start)=1, error in=w400) -> (refnum out=w394:refnum<file>, error out=w395:errorcluster)  [unwired: 1 in]
            n181 = Write to Text File(file (use dialog)=w394, text=w398, error in=w395) -> (refnum out=w397:refnum<file>, error out=w396:errorcluster)  [unwired: 1 in, 1 out]
            n182 = Flush File(refnum=w397, error in=w396) -> (error out=w399:errorcluster)  [unwired: 1 out]
          }
          frame #1 {
          }
        }
      }
      frame #3 {
        n183 = local read "measured data"() -> (w469:dbl[][])
        n184 = Insert Into Array(array=w469, new element=w468) -> (w467:dbl[][])  [unwired: 2 in]
        n185 = case shown="0, Default" w466 {
          tunnel: w467 -> [w485 w499]
          tunnel: "Y Axis" -> [w487 w498]
          tunnel: "X Axis" -> [w475 w497]
          frame #0 {
            n186 = Index Array(array=w485, index (col)=1 ("disabled index (col)")) -> (element=w480:dbl[])  [unwired: 1 in]
            n187 = Index Array(array=w485, index (col)=0 ("disabled index (col)")) -> (element=w479:dbl[])  [unwired: 1 in]
            n188 = Square(x=w480) -> (x^2=w482:dbl[])
            n189 = Square(x=w479) -> (x^2=w483:dbl[])
            n190 = Index Array(array=w485, index (col)=w487) -> (element=w474:dbl[])  [unwired: 1 in]
            n191 = Divide(x=w480, y=w479) -> (x/y=w471:dbl[])
            n192 = Add(x=w483, y=w482) -> (x+y=w481:dbl[])
            n193 = Inverse Tangent(1:w471) -> (0:w470:dbl[])
            n194 = Square Root(x=w481) -> (sqrt(x)=w472:dbl[])
            n195 = Divide(x=w470, y=3.141592653589793) -> (x/y=w477:dbl[])
            n196 = Multiply(x=w477, y=180) -> (x*y=w473:dbl[])
            n197 = case shown="\"B\", Default" w475 {
              tunnel: w474 -> [w490 w493]
              tunnel: w473 -> [_ w492]
              tunnel: w472 -> [w489 _]
              frame #0 {
                n198 = Bundle(w489, "measured data"=w490) -> (w488:cluster{dbl[], "measured data":dbl[]})  [unwired: 1 in]
                n199 = local write "XY Graph"(w488) -> ()
              }
              frame #1 {
                n200 = Bundle(w492, "measured data"=w493) -> (w491:cluster{dbl[], "measured data":dbl[]})  [unwired: 1 in]
                n201 = local write "XY Graph"(w491) -> ()
              }
            }
          }
          frame #1 {
            n202 = Index Array(array=w499, index (col)=w497) -> (element=w496:dbl[])  [unwired: 1 in]
            n203 = Index Array(array=w499, index (col)=w498) -> (element=w495:dbl[])  [unwired: 1 in]
            n204 = Bundle("measured data"=w496, "measured data"=w495) -> (w494:T2)  [unwired: 1 in]
            n205 = local write "XY Graph"(w494) -> ()
          }
        }
        n206 = local write "measured data"(w467) -> ()
      }
    }
    n207 = local read "Ramping Control"() -> (w257:u16)
    n208 = case shown="1" w257 {
      selector: w257 -> [w501 w516 w539 w543 w558]
      tunnel: w256 -> [_ w519 _ w546 w563]
      tunnel: w255 -> [_ w518 _ w545 w562]
      tunnel: [w500 w517 w538 w544 w561] -> w254
      tunnel: [w501 w516 w539 w543 w558] -> w252
      tunnel: w251 -> [_ _ _ w542 w560]
      tunnel: w250 -> [_ _ _ _ w557]
      tunnel: w249 -> [_ _ _ _ w556]
      tunnel: w248 -> [_ w508 _ _ _]
      tunnel: w247 -> [w500 w504 w538 w540 w555]
      frame #0 {
      }
      frame #1 {
        w511 = T9."HOLDING" ("y")
        n209 = local read "Number of lines"() -> (w505:i32)
        n210 = local read "Starting index"() -> (w507:i32)
        n211 = call <userlib>:"Get Ramping Mode.vi"("Communications Config"=w519, "error in"=w504) -> ("Ramping Mode"=w514:T10, "error out"=w515:T5)  [unwired: 1 out]
        n212 = call <userlib>:"Get Ramping Mode.vi"("Communications Config"=w518, "error in"=w515) -> ("Ramping Mode"=w513:T10, "error out"=w517:T5)  [unwired: 1 out]
        n213 = Less?(x=w507, y=w505) -> (x < y?=w506:bool)
        n214 = Equal?(x=w514, y=w511) -> (x = y?=w510:bool)
        n215 = Equal?(x=w513, y=w511) -> (x = y?=w509:bool)
        n216 = Compound Arithmetic op=AND(w510, w509) -> (w512:bool)
        n217 = case shown="True" w512 {
          tunnel: w508 -> [_ w523]
          tunnel: w506 -> [_ w522]
          tunnel: "Wait between \nVectors (ms)" -> [_ w521]
          tunnel: "Wait between \nVectors" -> [_ w520]
          frame #0 {
          }
          frame #1 {
            n218 = case shown="1" w523 {
              tunnel: w522 -> [_ w528]
              tunnel: w521 -> [_ w527]
              tunnel: w520 -> [_ w526]
              frame #0 {
                w525 = u16 2 items=["NEXT VECTOR", "RAMPING", "HOLDING", "PAUSE", "ZERO"] ("Ramping Control")
                n219 = local write "STATUS"("Holding at current vector. Set Ramping Mode to NEXT VECTOR to continue." ("STATUS")) -> ()
                n220 = local write "Ramping Control"(w525) -> ()
              }
              frame #1 {
                # "Go to NEXT VECTOR automatically"
                n221 = case shown="False" w528 {
                  tunnel: w527 -> [_ w532]
                  tunnel: w526 -> [_ w531]
                  frame #0 {
                    w530 = u16 2 items=["NEXT VECTOR", "RAMPING", "HOLDING", "PAUSE", "ZERO"] ("Ramping Control")
                    n222 = local write "STATUS"("Holding at current vector. Set Ramping Mode to NEXT VECTOR to continue." ("STATUS")) -> ()
                    n223 = local write "Ramping Control"(w530) -> ()
                  }
                  frame #1 {
                    n224 = stacked-sequence {
                      tunnel: w532 -> [w534 _]
                      tunnel: w531 -> [w533 _]
                      frame #0 {
                        n225 = case shown="True" w533 {
                          tunnel: w534 -> [_ w535]
                          frame #0 {
                          }
                          frame #1 {
                            n226 = Wait (ms)(milliseconds to wait=w535) -> ()  [unwired: 1 out]
                          }
                        }
                      }
                      frame #1 {
                        w537 = u16 0 items=["NEXT VECTOR", "RAMPING", "HOLDING", "PAUSE", "ZERO"] ("Ramping Control")
                        n227 = local write "Ramping Control"(w537) -> ()
                        n228 = local write "STATUS"("Go to NEXT VECTOR" ("STATUS")) -> ()
                      }
                    }
                  }
                }
              }
            }
          }
        }
      }
      frame #2 {
      }
      frame #3 {
        n229 = Not Equal?(x=w543, y=w542) -> (x != y?=w541:bool)
        n230 = case shown="False" w541 {
          tunnel: w546 -> [_ w554]
          tunnel: w545 -> [_ w553]
          tunnel: [w547 w551] -> w544
          tunnel: w540 -> [w547 w548]
          frame #0 {
          }
          frame #1 {
            w549 = u16 1 items=["RAMP", "PAUSE", "MANUAL UP", "MANUAL DOWN", "ZERO"] ("Ramping Mode")
            n231 = call <userlib>:"Set Ramping Mode.vi"("error in"=w548, "Ramping Mode"=w549, "Communications Config"=w554) -> ("error out"=w552:T5)
            n232 = call <userlib>:"Set Ramping Mode.vi"("error in"=w552, "Ramping Mode"=w549, "Communications Config"=w553) -> ("error out"=w551:T5)
            n233 = local write "STATUS"("All Programmers are PAUSED. Set Ramping Mode to NEXT VECTOR to continue." ("STATUS")) -> ()
          }
        }
      }
      frame #4 {
        n234 = Not Equal?(x=w558, y=w560) -> (x != y?=w559:bool)
        n235 = case shown="False" w559 {
          tunnel: w563 -> [_ w572]
          tunnel: w562 -> [_ w571]
          tunnel: [w564 w567] -> w561
          tunnel: w557 -> [_ w570]
          tunnel: w556 -> [_ w569]
          tunnel: w555 -> [w564 w565]
          frame #0 {
          }
          frame #1 {
            w566 = u16 4 items=["RAMP", "PAUSE", "MANUAL UP", "MANUAL DOWN", "ZERO"] ("Ramping Mode")
            n236 = local write "STATUS"("Zeroing vector." ("STATUS")) -> ()
            n237 = call <userlib>:"Set Ramping Mode.vi"("error in"=w565, "Ramping Mode"=w566, "Communications Config"=w572) -> ("error out"=w575:T5)
            n238 = call <userlib>:"Set Ramping Mode.vi"("error in"=w575, "Ramping Mode"=w566, "Communications Config"=w571) -> ("error out"=w568:T5)
            n239 = call <userlib>:"Set Current Ramp Rate.vi"("Communications Config"=w572, "Ramp Rate (A/sec)"=w570, "error in"=w568) -> ("error out"=w573:T5)  [unwired: 2 in]
            n240 = call <userlib>:"Set Current Ramp Rate.vi"("Communications Config"=w571, "Ramp Rate (A/sec)"=w569, "error in"=w573) -> ("error out"=w567:T5)  [unwired: 2 in]
          }
        }
      }
    }
    n241 = local read "Continue Execution?"() -> (w253:bool)
  }
  n242 = case shown="0, Default" w30 {
    tunnel: w26 -> [w578 _ _]
    tunnel: w24 -> [w577 w581 w582]
    tunnel: [w576 w580 w582] -> w31
    tunnel: w25 -> [_ w579 _]
    frame #0 {
      n243 = call <userlib>:"430_TCP_Close.vi"("error in (no error)"=w577, "connection ID"=w578) -> ("error out"=w576:errorcluster)  [unwired: 1 out]
    }
    frame #1 {
      n244 = call <userlib>:"430_RS232_Close.vi"("error in (no error)"=w581, "VISA resource name"=w579) -> ("error out"=w580:errorcluster)  [unwired: 1 in]
    }
    frame #2 {
    }
  }
  n245 = case shown="0, Default" w29 {
    tunnel: w28 -> [w585 _ _]
    tunnel: w31 -> [w584 w588 w589]
    tunnel: [w583 w587 w589] -> w21
    tunnel: w27 -> [_ w586 _]
    frame #0 {
      n246 = call <userlib>:"430_TCP_Close.vi"("error in (no error)"=w584, "connection ID"=w585) -> ("error out"=w583:errorcluster)  [unwired: 1 out]
    }
    frame #1 {
      n247 = call <userlib>:"430_RS232_Close.vi"("error in (no error)"=w588, "VISA resource name"=w586) -> ("error out"=w587:errorcluster)  [unwired: 1 in]
    }
    frame #2 {
    }
  }
  "error out" <- w21
  n248 = local read "Magnetic Field Units"() -> (w48:u16)
  n249 = local read "Coordinate System"() -> (w49:u16)
  n250 = while {
    tunnel: "Starting index" -> [w597]
    tunnel: w23 -> [w603]
    tunnel: w22 -> [w604]
    tunnel: w48 -> [w605]
    tunnel: w49 -> [w606]
    tunnel: w46 -> [w609]
    tunnel: "Max Ramp Rate - Y Axis (A/s)" -> [w593]
    tunnel: "Max Ramp Rate - Z Axis (A/s)" -> [w592]
    tunnel: "Magnitude Limit (kG)" -> [w594]
    tunnel: "User defined Ramp Rate (T/min)" -> [w591]
    tunnel: "User defined Ramp Rate (T/min)" -> [w590]
    i -> [w596]
    stop <- w598 continue-if-true
    n251 = local read "Field Values"() -> (w600:string[][])
    n252 = Add(x=w597, y=w596) -> (x+y=w595:i32)
    n253 = while "Wait for NEXT VECTOR setting by operator." {
      tunnel: [w613] -> w608
      tunnel: w609 -> [w613]
      stop <- w614 continue-if-true
      w612 = u16 0 items=["NEXT VECTOR", "RAMPING", "HOLDING", "PAUSE", "ZERO"] ("Ramping Control")
      n254 = local read "Ramping Control"() -> (w615:u16)
      n255 = Not Equal?(x=w612, y=w615) -> (x != y?=w614:bool)
    }
    n256 = stacked-sequence {
      tunnel: w595 -> [w617 _ w623 _]
      frame #0 {
        (unwired) -2
        n257 = Subtract(x=w617, y=2) -> (x-y=w620:i32)
        n258 = Bundle(w620, -2) -> (w618:cluster{i32, i32})  [unwired: 1 in]
        n259 = property on="Field Values" class="Tbl (strict)"("Active Cell:Active Cell"=w618) -> ()  [unwired: 2 in, 2 out]
      }
      frame #1 {
        n260 = local read "Normal color"() -> (w621:u32)
        n261 = property on="Field Values" class="Tbl (strict)"("Active Cell:Cell Background Color"=w621) -> ()  [unwired: 2 in, 2 out]
      }
      frame #2 {
        n262 = Decrement(x=w623) -> (x-1=w622:i32)
        n263 = Bundle(w622, -2) -> (w625:cluster{i32, i32})  [unwired: 1 in]
        n264 = property on="Field Values" class="Tbl (strict)"("Active Cell:Active Cell"=w625) -> ()  [unwired: 2 in, 2 out]
      }
      frame #3 {
        n265 = property on="Field Values" class="Tbl (strict)"("Active Cell:Cell Background Color"="Highlight color") -> ()  [unwired: 2 in, 2 out]
      }
    }
    n266 = Index Array(array=w600, index (row)=w595) -> (element=w607:string[])  [unwired: 1 in]
    n267 = local write "Starting index"(w595) -> ()
    n268 = Add(x=1, y=w595) -> (x+y=w610:i32)
    n269 = Number To Decimal String(number=w610) -> (decimal integer string=w599:string)  [unwired: 1 in]
    n270 = stacked-sequence {
      tunnel: [_ w651] -> w601
      tunnel: [_ w650] -> w602
      tunnel: w608 -> [_ w646]
      tunnel: w607 -> [_ w645]
      tunnel: w606 -> [_ w644]
      tunnel: w605 -> [_ w643]
      tunnel: w604 -> [_ w642]
      tunnel: w603 -> [_ w641]
      tunnel: w599 -> [_ w640]
      tunnel: w594 -> [_ w638]
      tunnel: w593 -> [_ w637]
      tunnel: w592 -> [_ w632]
      tunnel: w591 -> [_ w636]
      tunnel: w590 -> [_ w635]
      frame #0 {
        w630 = u16 1 items=["NEXT VECTOR", "RAMPING", "HOLDING", "PAUSE", "ZERO"] ("Ramping Control")
        n271 = local write "Ramping Control"(w630) -> ()
      }
      frame #1 {
        n272 = call <userlib>:"Set 2D Next Vector_entwurf.vi"("Coordinate System"=w644, "Magnetic Field Units"=w643, 3:"User defined Ramp Rate (T/min)"=w635, "Magnitude Limit (kG)"=w638, "Y-Axis Communications Config"=w642, "Input Vector"=w645, "Z-Axis Communications Config"=w641, 10:"User defined Ramp Rate (T/min)"=w636, "Max Ramp Rate - Y Axis (A/s)"=w637, "error in"=w646, "Max Ramp Rate - Z Axis (A/s)"=w632) -> ("Y-Axis Ramp Rate (T/min)"=→"Current Ramp Rate Y (T/min)":dbl, "Within Limits?"=w651:bool, "Ramp Rate along Vector (T/min)"=→"Ramp Rate along Vector (T/min)":dbl, "Z-Axis Ramp Rate (T/min)"=→"Current Ramp Rate Z (T/min)":dbl, "All Instruments Responded?"=w650:bool, "error out"=w639:T5)  [unwired: 3 in]
        n273 = Concatenate Strings("Ramping to field vector " ("STATUS"), w640, "..." ("STATUS")) -> (w647:string)
        n274 = local write "error in"(w639) -> ()
        n275 = local write "STATUS"(w647) -> ()
      }
    }
    n276 = case shown="True" w601 {
      tunnel: w602 -> [_ w628]
      frame #0 {
        n277 = local write "STATUS"("Vector magnitude limt or maximum coil current exceeded. Vector ignored. VI halted." ("STATUS")) -> ()
      }
      frame #1 {
        n278 = case shown="True" w628 {
          frame #0 {
            n279 = local write "STATUS"("Not all programmers responded. VI halted." ("STATUS")) -> ()
          }
          frame #1 {
          }
        }
      }
    }
    n280 = Compound Arithmetic op=AND(w602, w601) -> (w598:bool)
    n281 = local write "Continue Execution?"(w598) -> ()
  }
